vi "ASK MOD 3BpS.vi"() -> ()   [LabVIEW 2010]
panel:
  out "G1":dynamicdata(graph)
  out "G0":dynamicdata(graph)
  in  "Numérique":dbl
  in  "Tableau":bool[](array[boolean])
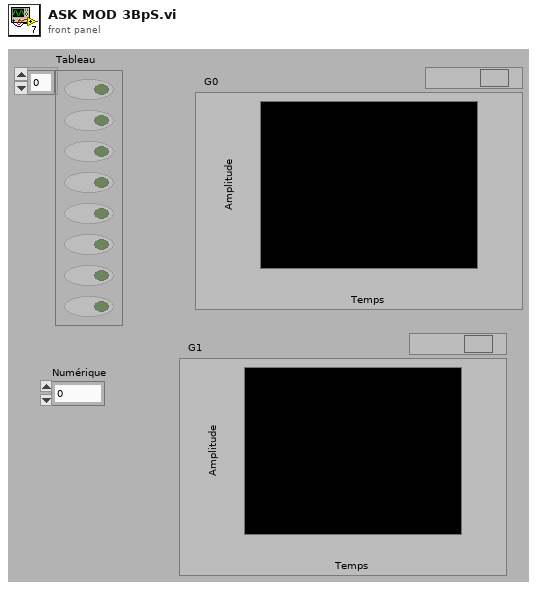
[diagram p1: front panel]
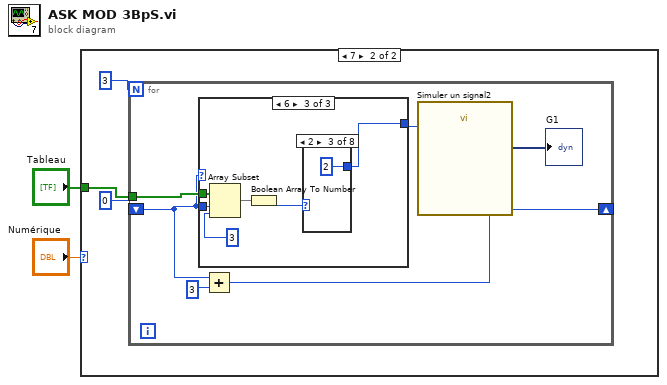
[diagram p0: block diagram]
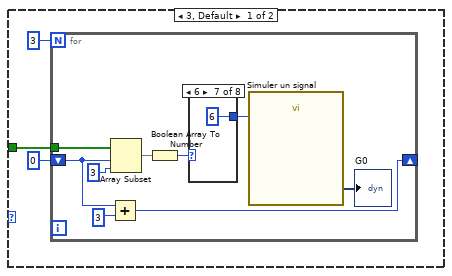
[diagram p2: hidden frame]
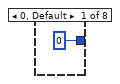
[diagram p3: hidden frame]
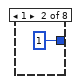
[diagram p4: hidden frame]
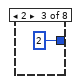
[diagram p5: hidden frame]
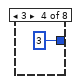
[diagram p6: hidden frame]
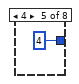
[diagram p7: hidden frame]
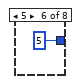
[diagram p8: hidden frame]
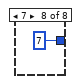
[diagram p9: hidden frame]
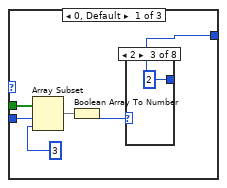
[diagram p10: hidden frame]
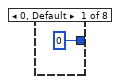
[diagram p11: hidden frame]
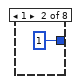
[diagram p12: hidden frame]
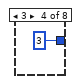
[diagram p13: hidden frame]
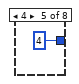
[diagram p14: hidden frame]
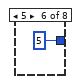
[diagram p15: hidden frame]
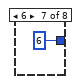
[diagram p16: hidden frame]
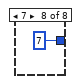
[diagram p17: hidden frame]
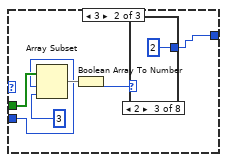
[diagram p18: hidden frame]
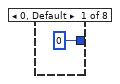
[diagram p19: hidden frame]
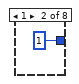
[diagram p20: hidden frame]
diagram:
  n1 = case shown="7" "Numérique" {
    tunnel: "Tableau" -> [w3 w23]
    frame 3, Default {
      n2 = for {
        N: 3 -> [_]
        shift-right: [w13] -> _
        shift-left: 0 -> [w11]
        tunnel: w3 -> [w8]
        n3 = Add(x=w11, y=3) -> (x+y=w13:i32)
        n4 = Array Subset(array=w8, index=w11, length=3 ("longueur")) -> (w12:bool[])
        n5 = Boolean Array To Number(Boolean array=w12) -> (number=w9:u32)
        n6 = case shown="6" w9 {
          tunnel: [0 1 2 3 4 ("longueur") 5 ("longueur") 6 ("longueur") 7 ("longueur")] -> w7
          frame 0, Default {
          }
          frame 1 {
          }
          frame 2 {
          }
          frame 3 {
          }
          frame 4 {
          }
          frame 5 {
          }
          frame 6 {
          }
          frame 7 {
          }
        }
        n7 = call "Simuler un signal"("Amplitude"=w7) -> ("Sinus"=→"G0":dynamicdata)  [unwired: 13 in, 1 out]
      }
    }
    frame 7 {
      n8 = for {
        N: 3 -> [_]
        shift-right: [w30] -> _
        shift-left: 0 -> [w26]
        tunnel: w23 -> [w29]
        n9 = case shown="6" w26 {
          tunnel: w29 -> [w34 w48 w62]
          tunnel: w26 -> [w33 w47 w61]
          tunnel: [w32 w46 w60] -> w27
          frame 0, Default {
            n10 = Array Subset(array=w34, index=w33, length=3 ("longueur")) -> (w37:bool[])
            n11 = Boolean Array To Number(Boolean array=w37) -> (number=w35:u32)
            n12 = case shown="2" w35 {
              tunnel: [0 1 2 3 4 ("longueur") 5 ("longueur") 6 ("longueur") 7 ("longueur")] -> w32
              frame 0, Default {
              }
              frame 1 {
              }
              frame 2 {
              }
              frame 3 {
              }
              frame 4 {
              }
              frame 5 {
              }
              frame 6 {
              }
              frame 7 {
              }
            }
          }
          frame 3 {
            n13 = Array Subset(array=w48, index=w47, length=3 ("longueur")) -> (w51:bool[])
            n14 = Boolean Array To Number(Boolean array=w51) -> (number=w49:u32)
            n15 = case shown="2" w49 {
              tunnel: [0 1 2 3 4 ("longueur") 5 ("longueur") 6 ("longueur") 7 ("longueur")] -> w46
              frame 0, Default {
              }
              frame 1 {
              }
              frame 2 {
              }
              frame 3 {
              }
              frame 4 {
              }
              frame 5 {
              }
              frame 6 {
              }
              frame 7 {
              }
            }
          }
          frame 6 {
            n16 = Array Subset(array=w62, index=w61, length=3 ("longueur")) -> (w65:bool[])
            n17 = Boolean Array To Number(Boolean array=w65) -> (number=w63:u32)
            n18 = case shown="2" w63 {
              tunnel: [0 1 2 7 4 ("longueur") 5 ("longueur") 6 ("longueur") 7 ("longueur")] -> w60
              frame 0, Default {
              }
              frame 1 {
              }
              frame 2 {
              }
              frame 3 {
              }
              frame 4 {
              }
              frame 5 {
              }
              frame 6 {
              }
              frame 7 {
              }
            }
          }
        }
        n19 = Add(x=w26, y=3) -> (x+y=w30:i32)
        n20 = call "Simuler un signal2"("Amplitude"=w27) -> ("Sinus"=→"G1":dynamicdata)  [unwired: 13 in, 1 out]
      }
    }
  }
